vi "Day 7 shift register.vi"() -> ()   [LabVIEW 2026]
panel:
  out "VALUE OF OUTPUT 4 ITERATION AGO":i32
  out "VALUE OF OUTPUT 3 ITERATION AGO":i32
  out "VALUE OF OUTPUT 2 ITERATION AGO":i32
  out "VALUE OF OUTPUT 1 ITERATION AGO":i32
  out "OUTPUT":i32
  out "iteration - output":i32
  out "output 2 - scalar (auto indexing off)":i32
  out "sum 2":i32
  out "iteration 2":i32
  out "Array 2":i32[](array[numeric])
  out "sum 1":i32
  out "Array 1":i32[](array[numeric])
  out "Output 1":i32
  out "iteration 1":i32
  out "Numeric":i32
  out "Numeric 2":i32
  out "output":i32
  out "n-1":dbl
  out "n - 4":dbl
  out "n - 3":dbl
  out "n-2":dbl
  out "Numeric":dbl
  # "Shift Register Example - 1"
  # "Shift Register Example - 2"
  # "Shift Register Example - 5"
  # "Shift Register Example - 4"
  # "Shift Register Example - 3"
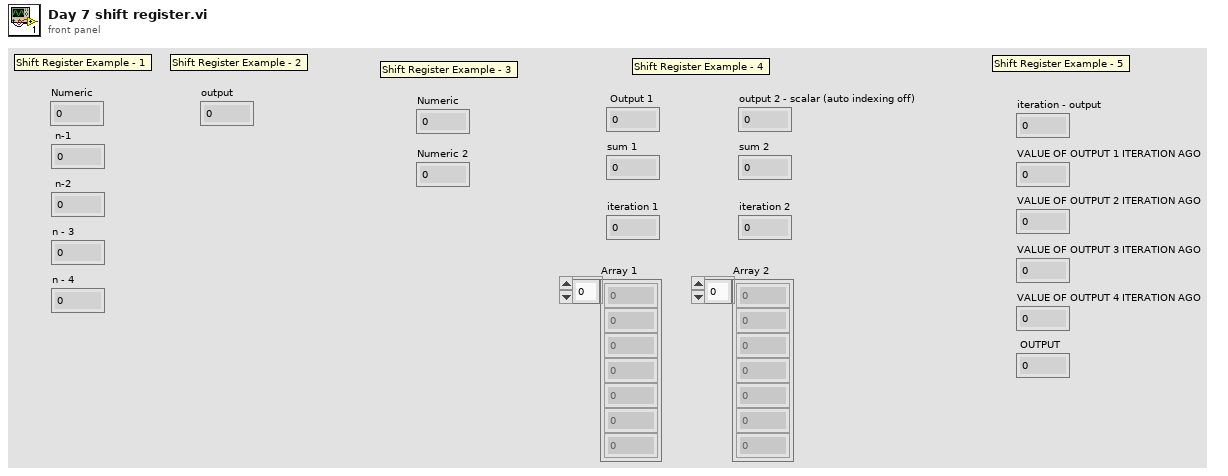
[diagram p1: front panel]
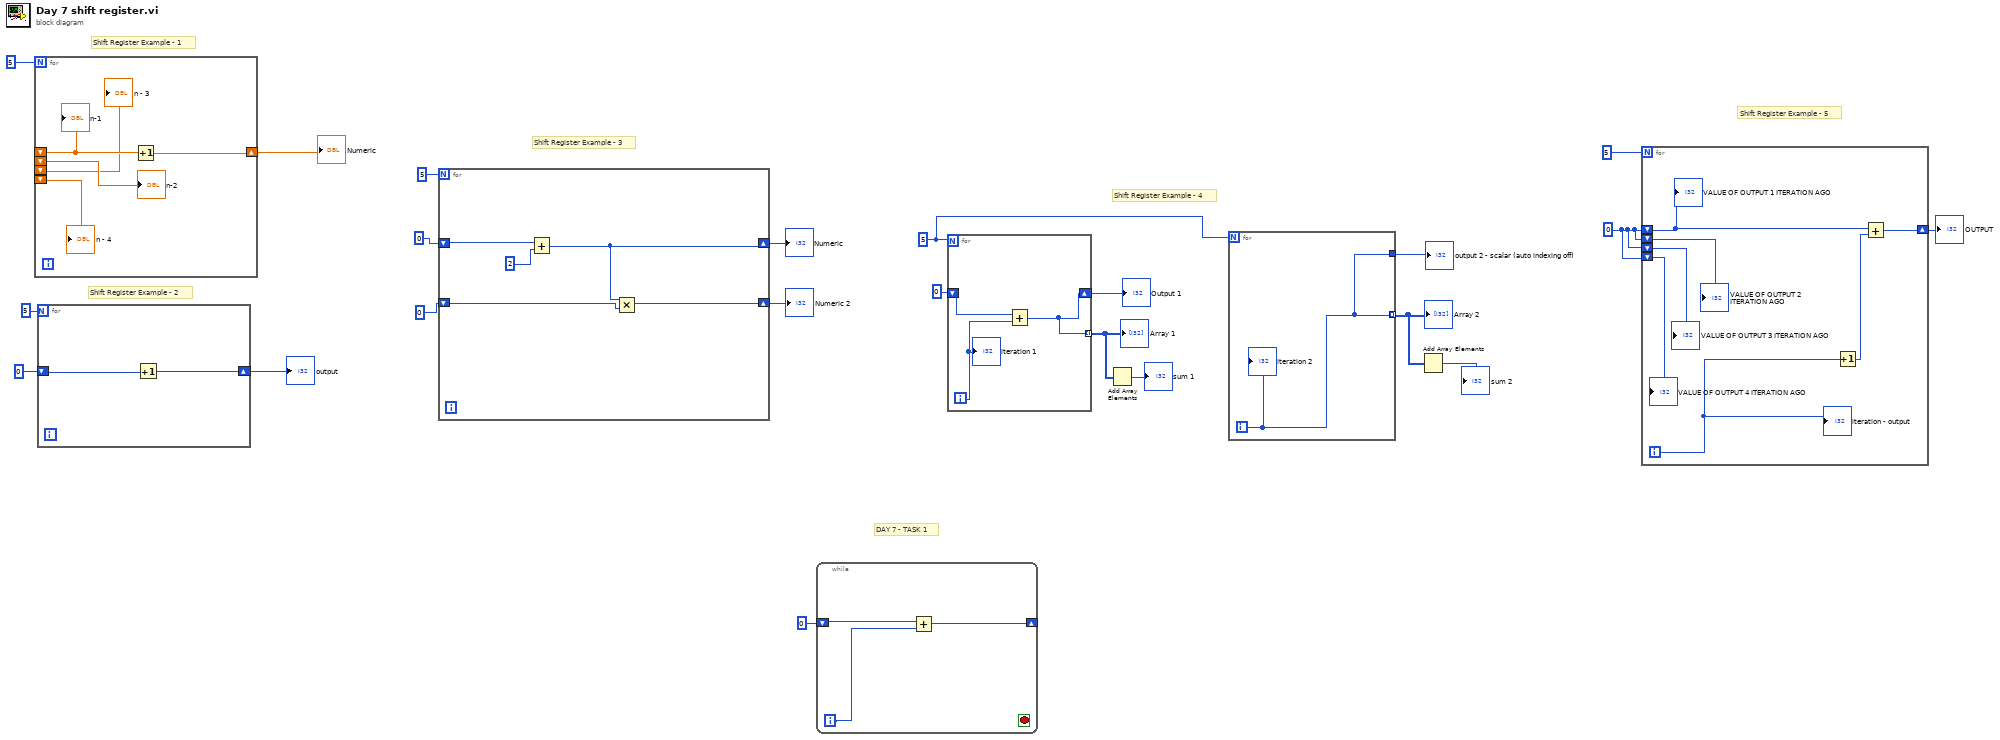
[diagram p0: block diagram]
diagram:
  w3 = 0
  w11 = 5
  # "DAY 7 - TASK 1"
  # "Shift Register Example - 5"
  # "Shift Register Example - 4"
  # "Shift Register Example - 3"
  # "Shift Register Example - 2"
  # "Shift Register Example - 1"
  n1 = for {
    N: 5 -> [_]
    shift-right: [w27] -> w22
    shift-left: _ -> [w28]
    shift-left: _ -> [w26]
    shift-left: _ -> [w25]
    shift-left: _ -> [w24]
    n2 = Increment(x=w28) -> (x+1=w27:dbl)
    "n-2" <- w26
    "n - 3" <- w25
    "n - 4" <- w24
    "n-1" <- w28
  }
  "Numeric" <- w22
  n3 = for {
    N: 5 -> [_]
    shift-right: [w29] -> w19
    shift-left: 0 -> [w30]
    n4 = Increment(x=w30) -> (x+1=w29:i32)
  }
  "output" <- w19
  n5 = for {
    N: 5 -> [_]
    shift-right: [w33] -> w14
    shift-left: 0 -> [w35]
    shift-right: [w31] -> w15
    shift-left: 0 -> [w32]
    n6 = Add(x=w35, y=2) -> (x+y=w33:i32)
    n7 = Multiply(x=w33, y=w32) -> (x*y=w31:i32)
  }
  "Numeric 2" <- w15
  "Numeric" <- w14
  n8 = while {
    shift-right: [w36] -> w1
    shift-left: 0 -> [w37]
    i -> [w38]
    stop <- w39 stop-if-true
    n9 = Add(x=w37, y=w38) -> (x+y=w36:i32)
  }
  n10 = for {
    N: w11 -> [_]
    shift-right: [w40] -> w13
    shift-left: 0 -> [w42]
    tunnel: [w40] -> w10 mode=indexing
    i -> [w41]
    n11 = Add(x=w42, y=w41) -> (x+y=w40:i32)
    "iteration 1" <- w41
  }
  "Output 1" <- w13
  "Array 1" <- w10
  n12 = Add Array Elements(numeric array=w10) -> (sum=→"sum 1":i32)
  n13 = for {
    N: w11 -> [_]
    tunnel: [w43] -> w8 mode=indexing
    tunnel: [w43] -> w6
    i -> [w43]
    "iteration 2" <- w43
  }
  "Array 2" <- w8
  "output 2 - scalar (auto indexing off)" <- w6
  n14 = Add Array Elements(numeric array=w8) -> (sum=→"sum 2":i32)
  n15 = for {
    N: 5 -> [_]
    shift-right: [w50] -> w4
    shift-left: w3 -> [w47]
    shift-left: w3 -> [w46]
    shift-left: w3 -> [w45]
    shift-left: w3 -> [w44]
    i -> [w48]
    n16 = Increment(x=w48) -> (x+1=w49:i32)
    n17 = Add(x=w47, y=w49) -> (x+y=w50:i32)
    "iteration - output" <- w48
    "VALUE OF OUTPUT 1 ITERATION AGO" <- w47
    "VALUE OF OUTPUT 2 ITERATION AGO" <- w46
    "VALUE OF OUTPUT 3 ITERATION AGO" <- w45
    "VALUE OF OUTPUT 4 ITERATION AGO" <- w44
  }
  "OUTPUT" <- w4
